vi "testSimulator.vi"(8 "error in (no error)":errorcluster) -> (0 "error out":errorcluster)   [LabVIEW 2018]
doc: "Test all test cases from simulator directory."
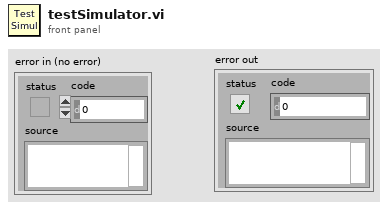
[diagram p1: front panel]
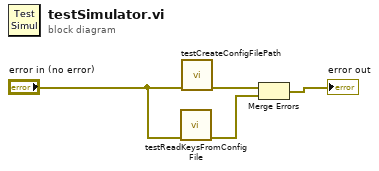
[diagram p0: block diagram]
diagram:
  n1 = call "testReadKeysFromConfigFile.vi"("error in (no error)"="error in (no error)") -> ("error out"=w1:errorcluster)  [unwired: 10 in]
  n2 = call "testCreateConfigFilePath.vi"("error in (no error)"="error in (no error)") -> ("error out"=w2:errorcluster)  [unwired: 10 in]
  n3 = Merge Errors(w2, w1) -> (→"error out":errorcluster)
